vi "MoveSailInEmergency.vi"(11 "ForceOnSails/Stays":dbl) -> ()   [LabVIEW 2012]
doc: "TODO: Make an algorithm that will move the sails into as low stress a position as possible, possibly perpendicular to the perceived wind. Try to be careful about letting the sails all the way out and getting them stuck. If this condition keeps on happening, the midbrain should go into Turtle Mode in DetermineBoatState.vi\n\nEric Schneider, Jan. 2014"
uses:
  Data/TypeDefs/Sail Set Suggestions.ctl
panel:
  out "EmergencySailSetting":T1 {"MainSailSuggestion" min=0.0 max=1.0; "JibSailSuggestion" min=0.0 max=1.0}
  in  "RelativeWindAngle":dbl
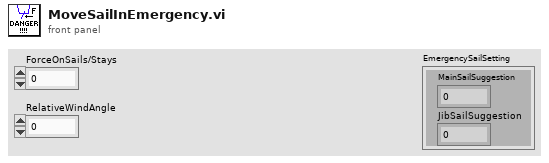
[diagram p1: front panel]
types:
  T1 = typedef "Sail Set Suggestions.ctl" = cluster{"MainSailSuggestion":dbl, "JibSailSuggestion":dbl}
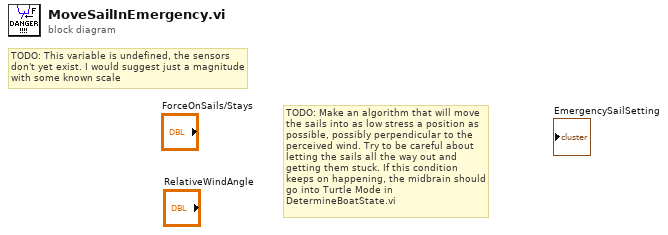
[diagram p0: block diagram]
diagram:
  # "TODO: Make an algorithm that will move the sails into as low stress a position as possible, possibly perpendicular to the perceived wind. Try to be careful about letting the sails all the way out and getting them stuck. If this condition keeps on happening, the midbrain should go into Turtle Mode in DetermineBoatState.vi"
  # "TODO: This variable is undefined, the sensors\ndon't yet exist. I would suggest just a magnitude\nwith some known scale"
